vi "Test Alarm.vi"(11 "Error in":errorcluster) -> (15 "Error out":errorcluster)   [LabVIEW 2020, in "Airplane Tests.lvlib"]
doc: "This VI validates the alarm tests"
uses:
  Airplane Tests.lvlib
  <vilib>/SLL Drona/APIs/Stimulus/ControlValue/SetValueAuto.vi
  <vilib>/SLL Drona/APIs/Assert/AssertControlValue/Equal.vi
  <vilib>/SLL Drona/APIs/Assert/AssertControlValue/Less.vi
  <vilib>/SLL Drona/APIs/Stimulus/VI/CloseVI.vi
  <vilib>/addons/_JKI Toolkits/Caraya/classes/Test/Test.lvclass
  <vilib>/SLL Drona/Drona.lvlib
  <vilib>/SLL Drona/APIs/Stimulus/ControlValue/ControlValue.lvlib
  <vilib>/SLL Drona/APIs/Assert/AssertControlValue/AssertControlValue.lvlib
  <vilib>/SLL Drona/APIs/Stimulus/VI/VI.lvlib
panel:
  # "ALARM TEST"
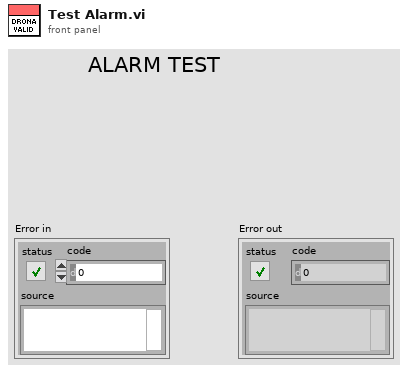
[diagram p1: front panel]
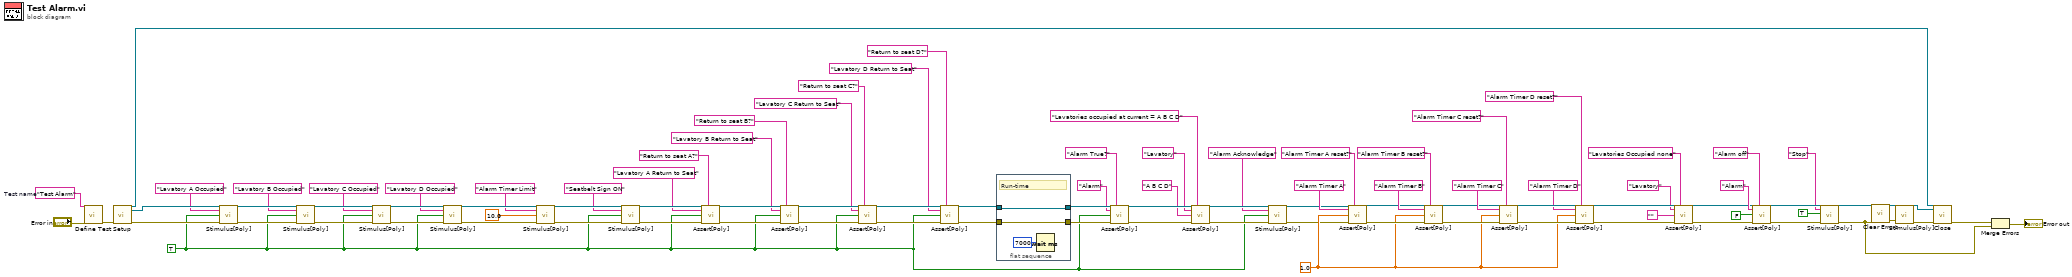
[diagram p0: block diagram]
diagram:
  w23 = 1.0
  (unwired) 10.0
  w49 = TRUE
  w6 = "Test Alarm"  # Test name
  n1 = call <vilib>:"Define Test.vi"("error in (no error)"="Error in", "Label (VI Title)"=w6) -> ("error out"=w92:errorcluster)  [unwired: 8 in, 1 out]
  n2 = call <vilib>:"Setup.vi"("error in"=w92) -> ("Application Ref"=w7:refnum<vi>, "VI Reference Out"=w90:refnum<vi>, "error out"=w91:errorcluster)  [unwired: 12 in]
  n3 = call-poly <vilib>:"Stimulus[Poly].vi"("VI Reference In"=w90, "Control Path"="Lavatory A Occupied", "Value (Signaling)"=w49, "error in"=w91) -> ("VI Reference Out"=w87:refnum<vi>, "error out"=w88:errorcluster)  [unwired: 10 in]
  n4 = call-poly <vilib>:"Stimulus[Poly].vi"("VI Reference In"=w87, "Control Path"="Lavatory B Occupied", "Value (Signaling)"=w49, "error in"=w88) -> ("VI Reference Out"=w86:refnum<vi>, "error out"=w89:errorcluster)  [unwired: 10 in]
  n5 = call-poly <vilib>:"Stimulus[Poly].vi"("VI Reference In"=w86, "Control Path"="Lavatory C Occupied", "Value (Signaling)"=w49, "error in"=w89) -> ("VI Reference Out"=w85:refnum<vi>, "error out"=w84:errorcluster)  [unwired: 10 in]
  n6 = call-poly <vilib>:"Stimulus[Poly].vi"("VI Reference In"=w85, "Control Path"="Lavatory D Occupied", "Value (Signaling)"=w49, "error in"=w84) -> ("VI Reference Out"=w79:refnum<vi>, "error out"=w78:errorcluster)  [unwired: 10 in]
  n7 = call-poly <vilib>:"Stimulus[Poly].vi"("VI Reference In"=w79, "Control Path"="Alarm Timer Limit", "Value (Signaling)"=10.0, "error in"=w78) -> ("VI Reference Out"=w76:refnum<vi>, "error out"=w77:errorcluster)  [unwired: 10 in]
  n8 = call-poly <vilib>:"Stimulus[Poly].vi"("VI Reference In"=w76, "Control Path"="Seatbelt Sign ON", "Value (Signaling)"=w49, "error in"=w77) -> ("VI Reference Out"=w69:refnum<vi>, "error out"=w73:errorcluster)  [unwired: 10 in]
  n9 = call-poly <vilib>:"Assert[Poly].vi"("VI Reference In"=w69, "Test Label"="Return to seat A?" ("Label"), "Control Path"="Lavatory A Return to Seat", "Control Value"=w49, "Error In"=w73) -> ("VI Reference Out"=w68:refnum<vi>, "Error Out"=w72:errorcluster)  [unwired: 9 in]
  n10 = call-poly <vilib>:"Assert[Poly].vi"("VI Reference In"=w68, "Test Label"="Return to seat B?" ("Label"), "Control Path"="Lavatory B Return to Seat", "Control Value"=w49, "Error In"=w72) -> ("VI Reference Out"=w67:refnum<vi>, "Error Out"=w71:errorcluster)  [unwired: 9 in]
  n11 = call-poly <vilib>:"Assert[Poly].vi"("VI Reference In"=w67, "Test Label"="Return to seat C?" ("Label"), "Control Path"="Lavatory C Return to Seat", "Control Value"=w49, "Error In"=w71) -> ("VI Reference Out"=w66:refnum<vi>, "Error Out"=w70:errorcluster)  [unwired: 9 in]
  n12 = call-poly <vilib>:"Assert[Poly].vi"("VI Reference In"=w66, "Test Label"="Return to seat D?" ("Label"), "Control Path"="Lavatory D Return to Seat", "Control Value"=w49, "Error In"=w70) -> ("VI Reference Out"=w58:refnum<vi>, "Error Out"=w61:errorcluster)  [unwired: 9 in]
  n13 = flat-sequence {
    tunnel: [w95] -> w60
    tunnel: w61 -> [w95]
    tunnel: [w93] -> w59
    tunnel: w58 -> [w93]
    frame #0 {
      # "Run-time"
      n14 = Wait (ms)(milliseconds to wait=u32 7000) -> ()  [unwired: 1 out]
    }
  }
  n15 = call-poly <vilib>:"Assert[Poly].vi"("VI Reference In"=w59, "Test Label"="Alarm True?" ("Control Path"), "Control Path"="Alarm", "Control Value"=w49, "Error In"=w60) -> ("VI Reference Out"=w55:refnum<vi>, "Error Out"=w56:errorcluster)  [unwired: 9 in]
  n16 = call-poly <vilib>:"Assert[Poly].vi"("VI Reference In"=w55, "Test Label"="Lavatories occupied at current = A B C D" ("Control Path"), "Control Path"="Lavatory", "Control Value"="A B C D" ("Control Path"), "Error In"=w56) -> ("VI Reference Out"=w51:refnum<vi>, "Error Out"=w52:errorcluster)  [unwired: 9 in]
  n17 = call-poly <vilib>:"Stimulus[Poly].vi"("VI Reference In"=w51, "Control Path"="Alarm Acknowledge", "Value (Signaling)"=w49, "error in"=w52) -> ("VI Reference Out"=w15:refnum<vi>, "error out"=w22:errorcluster)  [unwired: 10 in]
  n18 = call-poly <vilib>:"Assert[Poly].vi"("VI Reference In"=w15, "Test Label"="Alarm Timer A reset?" ("Control Path"), "Control Path"="Alarm Timer A", "Control Value"=w23, "Error In"=w22) -> ("VI Reference Out"=w41:refnum<vi>, "Error Out"=w48:errorcluster)  [unwired: 9 in]
  n19 = call-poly <vilib>:"Assert[Poly].vi"("VI Reference In"=w41, "Test Label"="Alarm Timer B reset?" ("Control Path"), "Control Path"="Alarm Timer B", "Control Value"=w23, "Error In"=w48) -> ("VI Reference Out"=w40:refnum<vi>, "Error Out"=w47:errorcluster)  [unwired: 9 in]
  n20 = call-poly <vilib>:"Assert[Poly].vi"("VI Reference In"=w40, "Test Label"="Alarm Timer C reset?" ("Control Path"), "Control Path"="Alarm Timer C", "Control Value"=w23, "Error In"=w47) -> ("VI Reference Out"=w39:refnum<vi>, "Error Out"=w46:errorcluster)  [unwired: 9 in]
  n21 = call-poly <vilib>:"Assert[Poly].vi"("VI Reference In"=w39, "Test Label"="Alarm Timer D reset?" ("Control Path"), "Control Path"="Alarm Timer D", "Control Value"=w23, "Error In"=w46) -> ("VI Reference Out"=w38:refnum<vi>, "Error Out"=w45:errorcluster)  [unwired: 9 in]
  n22 = call-poly <vilib>:"Assert[Poly].vi"("VI Reference In"=w38, "Test Label"="Lavatories Occupied none" ("Control Path"), "Control Path"="Lavatory", "Control Value"="", "Error In"=w45) -> ("VI Reference Out"=w32:refnum<vi>, "Error Out"=w33:errorcluster)  [unwired: 9 in]
  n23 = call-poly <vilib>:"Assert[Poly].vi"("VI Reference In"=w32, "Test Label"="Alarm off" ("Control Path"), "Control Path"="Alarm", "Control Value"=FALSE, "Error In"=w33) -> ("VI Reference Out"=w13:refnum<vi>, "Error Out"=w14:errorcluster)  [unwired: 9 in]
  n24 = call-poly <vilib>:"Stimulus[Poly].vi"("VI Reference In"=w13, "Control Path"="Stop", "Value (Signaling)"=TRUE, "error in"=w14) -> ("VI Reference Out"=w10:refnum<vi>, "error out"=w4:errorcluster)  [unwired: 10 in]
  n25 = call <vilib>:"Clear Errors.vi"("error in (no error)"=w4) -> ("error out"=w5:errorcluster)  [unwired: 5 in, 1 out]
  n26 = call-poly <vilib>:"Stimulus[Poly].vi"("VI Reference In"=w10, "error in"=w5) -> ("VI Reference Out"=w8:refnum<vi>, "error out"=w9:errorcluster)  [unwired: 12 in]
  n27 = call <vilib>:"Close.vi"("Application Ref"=w7, "VI Reference"=w8, "error in"=w9) -> ("error out"=w2:errorcluster)  [unwired: 12 in]
  n28 = Merge Errors(w2, w4) -> (→"Error out":errorcluster)
